vi "Send message.vi"(8 "error in (no error)":errorcluster, 10 "message":string, 11 "Server in":refnum<class "TCP-Server.lvclass">) -> (0 "error out":errorcluster, 3 "Server out":refnum<class "TCP-Server.lvclass">)   [LabVIEW 2018, in "TCP-Server.lvclass"]
uses:
  TCP-Server.lvclass
  TCP-Server.lvclass/TCP-Server.ctl
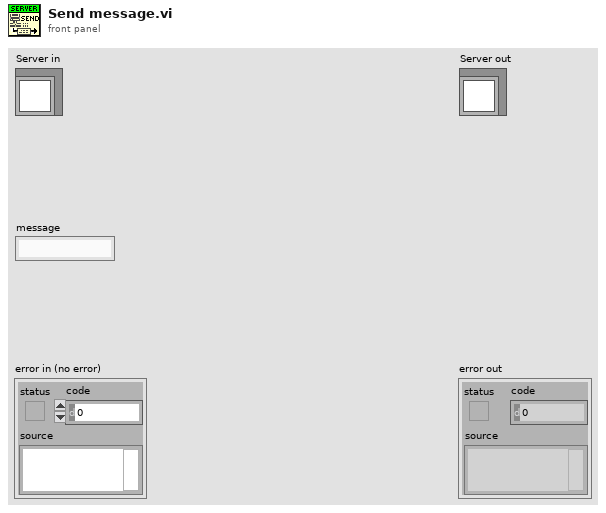
[diagram p1: front panel]
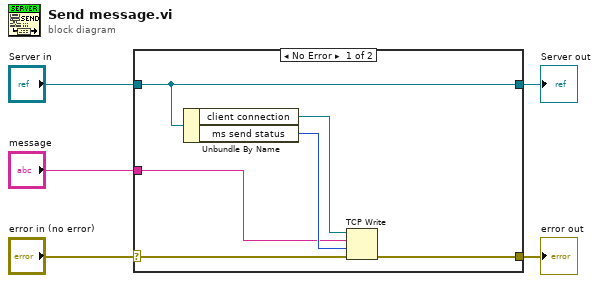
[diagram p0: block diagram]
diagram:
  n1 = case shown="No Error" "error in (no error)" {
    selector: "error in (no error)" -> [w9 w12]
    tunnel: [w8 w12] -> w4
    tunnel: [w11 w13] -> w2
    tunnel: "Server in" -> [w11 w13]
    tunnel: "message" -> [w6 _]
    frame No Error {
      n2 = Unbundle By Name(w11) -> ("client connection"=w10:refnum<k5>, "ms send status"=w7:i32)
      n3 = TCP Write(connection ID=w10, data in=w6, error in (no error)=w9, 9:w7) -> (error out=w8:errorcluster)  [unwired: 2 out]
    }
    frame Error {
    }
  }
  "error out" <- w4
  "Server out" <- w2
